vi "Team Selection UI.vi"(7 "Dev Team":refnum<class "Team.lvclass">) -> (1 "Cancelled":bool, 3 "Team":refnum<class "Team.lvclass">)   [LabVIEW 2020, in "SB App.lvlib" / "SB App.lvclass"]
uses:
  SB App.lvclass
  SquareBattle/Team/Team.lvclass
  c5aea009-a846-4be9-b2bb-55857650a0a4.vi
  <vilib>/Comparison/Equal/Equal Functor/Equal Functor.lvclass
panel:
  out "Available Teams":refnum<class "Team.lvclass">[](array[class])
  in  "Cancel Button":bool
  in  "OK Button":bool
  in  "Selected Team":i32(listbox)
  # "Select Team to add to game:"
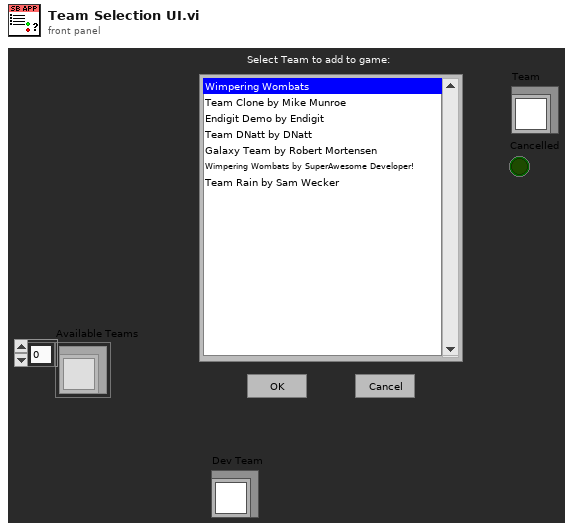
[diagram p1: front panel]
types:
  T1 = enum32{"Invalid", "Standard", "Closed", "Hidden", "Minimized", "Maximized"}
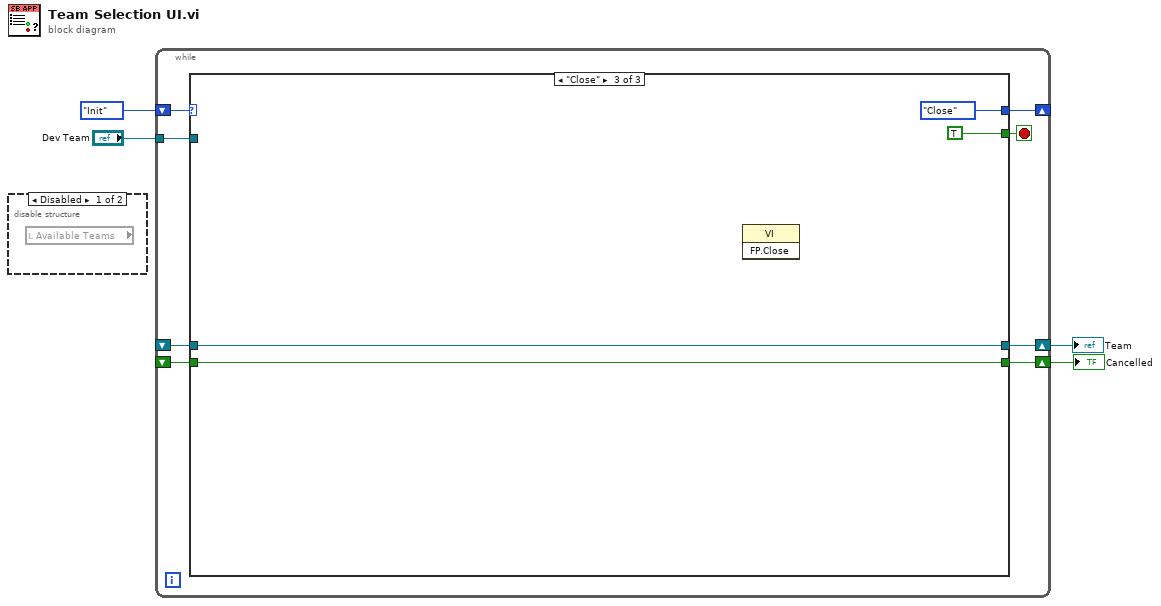
[diagram p0: block diagram]
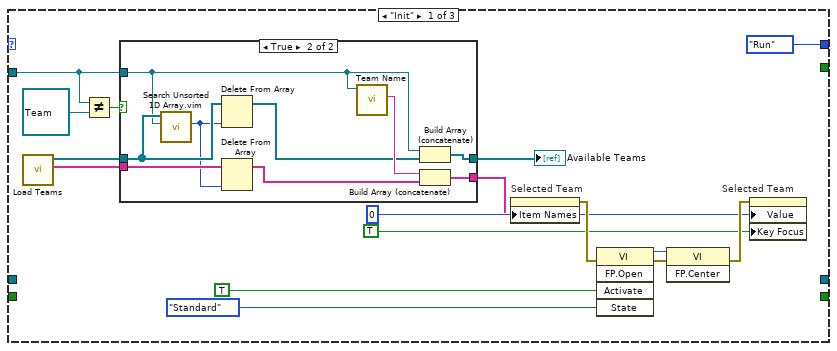
[diagram p3: hidden frame]
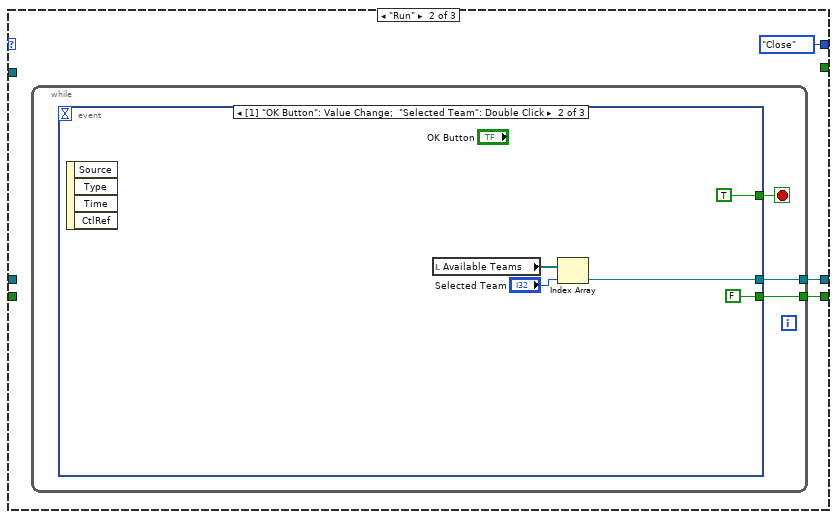
[diagram p5: hidden frame]
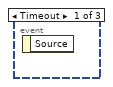
[diagram p6: hidden frame]
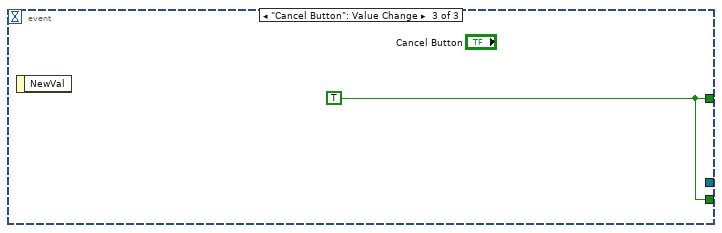
[diagram p7: hidden frame]
diagram:
  n1 = disable-structure shown="Disabled" {
    frame Disabled {
      n2 = local read "Available Teams"() -> ()  [unwired: 1 out]
    }
    frame Enabled {
    }
  }
  n3 = while {
    shift-right: [w11] -> _
    shift-left: enum16{"Init", "Run", "Close"}."Init" ("Basic UI State") -> [w12]
    shift-right: [w9] -> w3
    shift-left: _ -> [w8]
    shift-right: [w7] -> w2
    shift-left: _ -> [w6]
    tunnel: "Dev Team" -> [w5]
    stop <- w10 stop-if-true
    n4 = case shown="\"Close\"" w12 {
      tunnel: [enum16{"Init", "Run", "Close"}."Run" ("Basic UI State") enum16{"Init", "Run", "Close"}."Close" ("Basic UI State") enum16{"Init", "Run", "Close"}."Close" ("Basic UI State")] -> w11
      tunnel: [_ _ TRUE] -> w10
      tunnel: [_ w41 w53] -> w9
      tunnel: w8 -> [_ _ w53]
      tunnel: [_ w40 w52] -> w7
      tunnel: w6 -> [_ _ w52]
      tunnel: w5 -> [w16 _ _]
      frame "Init" {
        n5 = call "Load Teams.vi"() -> ("Names"=w15:string[], "Available Teams"=w18:refnum<class "Team.lvclass">[])  [unwired: 10 in]
        n6 = Not Equal?(x=w16, y=refnum<class "Team.lvclass"> refnum) -> (x != y?=w17:bool)
        n7 = case shown="True" w17 {
          tunnel: w18 -> [w30 w39]
          tunnel: w16 -> [_ w35]
          tunnel: w15 -> [w29 w34]
          tunnel: [w30 w37] -> w14
          tunnel: [w29 w36] -> w13
          frame False {
          }
          frame True {
            n8 = call "Search Unsorted 1D Array.vim"("element"=w35, "unsorted 1D array"=w39) -> ("index of element"=w33:i32)  [unwired: 9 in]
            n9 = Delete From Array(array=w39, index=w33) -> (array with subset deleted=w31:refnum<class "Team.lvclass">[])  [unwired: 1 in, 1 out]
            n10 = Delete From Array(array=w34, index=w33) -> (array with subset deleted=w32:string[])  [unwired: 1 in, 1 out]
            n11 = call-dynamic "Team Name.vi"("Team in"=w35) -> ("Team Name"=w38:string)  [unwired: 10 in]
            n12 = Build Array (concatenate)(w35, w31) -> (w37:refnum<class "Team.lvclass">[])
            n13 = Build Array (concatenate)(w38, w32) -> (w36:string[])
          }
        }
        "Available Teams" <- w14
        n14 = property on="Selected Team" class="LstBox (strict)"("Item Names"=w13) -> (error out=w23:errorcluster)  [unwired: 2 in, 1 out]
        n15 = invoke class="VI" method="FP.Open"(error in=w23, "Activate"=TRUE ("Activate?"), "State"=T1."Standard") -> (reference out=w24:refnum<vi>, error out=w22:errorcluster)  [unwired: 2 in, 3 out]
        n16 = invoke class="VI" method="FP.Center"(reference=w24, error in=w22) -> (error out=w28:errorcluster)  [unwired: 1 in, 2 out]
        n17 = property on="Selected Team" class="LstBox (strict)"(error in=w28, "Value"=0 ("Team"), "Key Focus"=TRUE) -> ()  [unwired: 1 in, 2 out]
      }
      frame "Run" {
        n18 = while {
          tunnel: [w45] -> w41
          tunnel: [w43] -> w40
          stop <- w44 stop-if-true
          n19 = event shown="[1] \"OK Button\": Value Change;  \"Selected Team\": Double Click" {
            selector: _ -> [_ _ _]
            dyn-events: _ -> [_ _ _]
            timeout: _ -> [_ _ _]
            tunnel: [_ w48 _] -> w45
            tunnel: [_ TRUE w51] -> w44
            tunnel: [_ FALSE w51] -> w43
            event Timeout {
              n20 = event-data() -> ()  [unwired: 1 in, 1 out]
            }
            event "OK Button": Value Change; "Selected Team": Double Click {
              n21 = event-data() -> ()  [unwired: 1 in, 4 out]
              n22 = local read "Available Teams"() -> (w50:refnum<class "Team.lvclass">[])
              n23 = Index Array(array=w50, index="Selected Team") -> (element=w48:refnum<class "Team.lvclass">)
            }
            event "Cancel Button": Value Change {
              w51 = TRUE
              n24 = event-data() -> ()  [unwired: 1 in, 1 out]
            }
          }
        }
      }
      frame "Close" {
        n25 = invoke class="VI" method="FP.Close"() -> ()  [unwired: 3 in, 3 out]
      }
    }
  }
  "Team" <- w3
  "Cancelled" <- w2
